vi "Callback Change P.vi"(6 "Variant":variant, 8 "error in (no error)":errorcluster, 9 "Old Values":string[][](array[string]), 10 "object ref in":T1, 11 "Table Change":T2) -> (0 "error out":errorcluster)   [LabVIEW 2015, in "PID Module 2 editor node.lvclass"]
doc: "This VI gets called automatically when changes are made to the 'Tag' column of the table and must handle changes appropriately. Register this callback using the appropriate 'Define Column' VI from the Table API."
uses:
  PID Module 2 editor node.lvclass
  <vilib>/NI/DCAF/Tag Editor Core/Table API/Table Manager/Cell Change.ctl
  <vilib>/NI/DCAF/Tag Editor Core/Table API/Table Manager/object ref.ctl
  <vilib>/NI/DCAF/Tag Editor Core/Configuration Editor/Classes/Engine Parent/Engine Parent Editor Node.lvclass
  <vilib>/NI/DCAF/Tag Editor Core/Configuration Editor/Classes/Module editor node/module editor node.lvclass
  <vilib>/NI/Tag Bus Module Framework/channel/TBM channel.lvclass
  <vilib>/NI/Tag Bus/tag/tag descriptor.lvclass/tag descriptor.ctl
  module/configuration/PID Module 2 configuration.lvclass
  module/configuration/PID Module 2 configuration.lvclass/PID Module 2 configuration.ctl
  module/configuration/Get Line Name.vi
  <vilib>/NI/Tag Bus Module Framework/module configuration/FindDuplicate.vi
  <vilib>/Utility/error.llb/Error Cluster From Error Code.vi
  <vilib>/NI/Tag Bus/tag/tag descriptor.lvclass
  <vilib>/NI/DCAF/Tag Editor Core/Table API/Table Manager.lvlib
  <vilib>/NI/DCAF/Tag Editor Core/Table API/Table Manager/Table Manager.lvclass
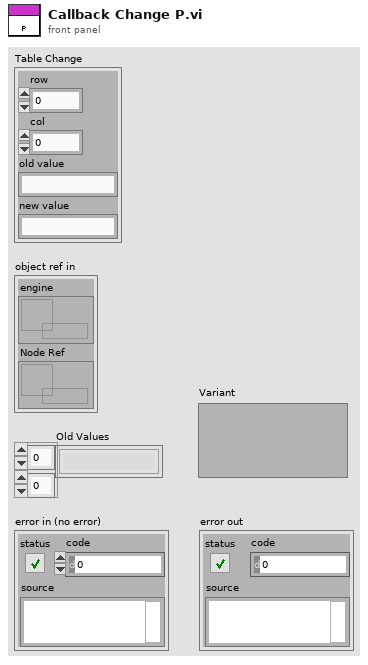
[diagram p1: front panel]
types:
  T1 = typedef "Table Manager.lvlib/Table Manager.lvclass/object ref.ctl" = cluster{"engine":refnum<data-value>, "Node Ref":refnum<data-value>}
  T2 = typedef "Table Manager.lvlib/Cell Change.ctl" = cluster{"row":i32, "col":i32, "old value":string, "new value":string}
  T3 = typedef "PID Module 2 configuration.lvclass/Line.ctl" = cluster{"PID ID":string, "Setpoint":refnum<class "TBM channel.lvclass">, "Variable":refnum<class "TBM channel.lvclass">, "Output":refnum<class "TBM channel.lvclass">, "Output High":refnum<class "TBM channel.lvclass">, "Output Low":refnum<class "TBM channel.lvclass">, "P":refnum<class "TBM channel.lvclass">, "I":refnum<class "TBM channel.lvclass">, "D":refnum<class "TBM channel.lvclass">}
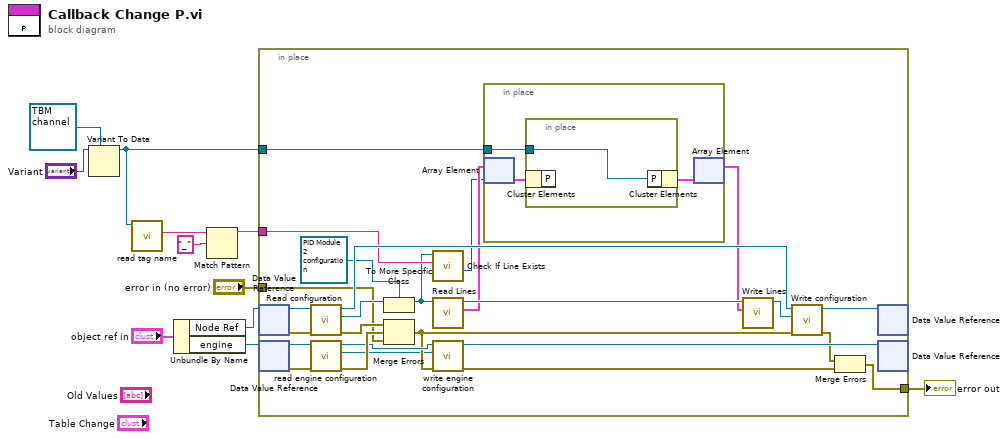
[diagram p0: block diagram]
diagram:
  n1 = Variant To Data(type=refnum<class "TBM channel.lvclass"> refnum ("output"), Variant="Variant") -> (data=w4:refnum<class "TBM channel.lvclass">)  [unwired: 1 in, 1 out]
  n2 = call <vilib>:"read tag name.vi"("system tag in"=w4) -> ("name"=w3:string)  [unwired: 8 in, 2 out]
  n3 = Unbundle By Name("object ref in") -> ("Node Ref"=w8:refnum<data-value>, "engine"=w7:refnum<data-value>)
  n4 = Match Pattern(string=w3, regular expression="_") -> (before substring=w1:string)  [unwired: 1 in, 3 out]
  n5 = in-place {
    in-place-border: [w29] -> w11
    in-place-border: "error in (no error)" -> [w22]
    in-place-border: w4 -> [w12]
    in-place-border: w1 -> [w19]
    n6 = in-place-dvr #1(w8) -> (w26:refnum<class "module editor node.lvclass">, w28:errorcluster)
    n7 = in-place-dvr #2(w7) -> (w36:refnum<class "Engine Parent Editor Node.lvclass">, w37:errorcluster)
    n8 = call-dynamic "Read configuration.vi"("error in"=w28, "NISE_CEF_serializable node in"=w26) -> ("error out"=w27:errorcluster, "configuration"=w24:refnum<class "NISE_CEF_serializable configuration.lvclass">, "NISE_CEF_serializable node out"=w25:refnum<class "module editor node.lvclass">)  [unwired: 7 in]
    n9 = call <vilib>:"read engine configuration.vi"("error in"=w37, "Engine Parent Editor Node in"=w36) -> ("error out"=w33:errorcluster, "engine configuration"=w21:refnum<class "engine configuration.lvclass">, "Engine Parent Editor Node out"=w32:refnum<class "Engine Parent Editor Node.lvclass">)  [unwired: 7 in]
    n10 = To More Specific Class(target class=refnum<class "PID Module 2 configuration.lvclass"> refnum ("tag bus configurable plugin module configuration"), reference=w24) -> (specific class reference=w16:refnum<class "PID Module 2 configuration.lvclass">)  [unwired: 1 in, 1 out]
    n11 = Merge Errors(w27, w33, w22) -> (w23:errorcluster)
    n12 = call-dynamic "Check If Line Exists.vi"("Name to Locate"=w19, "PID Module 2 configuration in"=w16) -> ("Index"=w14:i32)  [unwired: 5 in, 4 out]
    n13 = call "Read Lines.vi"("PID Module 2 configuration in"=w16) -> ("Lines"=w15:T3[], "PID Module 2 configuration out"=w17:refnum<class "PID Module 2 configuration.lvclass">)  [unwired: 8 in, 1 out]
    n14 = call <vilib>:"write engine configuration.vi"("error in"=w23, "engine configuration"=w21, "Engine Parent Editor Node in"=w32) -> ("error out"=w31:errorcluster, "Engine Parent Editor Node out"=w35:refnum<class "Engine Parent Editor Node.lvclass">)  [unwired: 7 in]
    n15 = in-place {
      in-place-border: w12 -> [w38]
      n16 = in-place-array #3(w15, w14) -> (w40:T3)
      n17 = in-place {
        in-place-border: w38 -> [w41]
        n18 = in-place-cluster #4(w40) -> ()  [unwired: 1 out]
        n19 = in-place-cluster #4("P"=w41) -> (w39:T3)
      }
      n20 = in-place-array #3(w39) -> (w13:T3[])  [unwired: 1 out]
    }
    n21 = call "Write Lines.vi"("Lines"=w13, "PID Module 2 configuration in"=w17) -> ("PID Module 2 configuration out"=w18:refnum<class "PID Module 2 configuration.lvclass">)  [unwired: 8 in, 1 out]
    n22 = call-dynamic "Write configuration.vi"("error in"=w23, "configuration"=w18, "NISE_CEF_serializable node in"=w25) -> ("error out"=w30:errorcluster, "NISE_CEF_serializable node out"=w34:refnum<class "module editor node.lvclass">)  [unwired: 7 in]
    n23 = Merge Errors(w30, w31) -> (w29:errorcluster)
    n24 = in-place-dvr #1(w34) -> ()  [unwired: 2 out]
    n25 = in-place-dvr #2(w35) -> ()  [unwired: 2 out]
  }
  "error out" <- w11
